vi "rx_trig_capt.vi"(7 "number of samples":i64=-1, 8 "error in (no error)":errorcluster, 9 "reference\nposition":dbl format="%0.2f", 10 "trigger level":dbl format="%0.2f", 11 "session handle":refnum<k15>) -> (0 "error out":errorcluster, 1 "packet found":bool, 2 "IQ Waveform":cluster{"t0":dbl, "dt":dbl, "Y":cdb[]}, 3 "session handle out":refnum<k15>)   [LabVIEW 2012, in "gds_hw_config.lvlib"]
uses:
  <instrlib>/niUSRP/niUSRP Fetch Rx Data (CDB Cluster).vi
  gds_hw_config.lvlib
  <vilib>/Analysis/NI_AALPro.lvlib
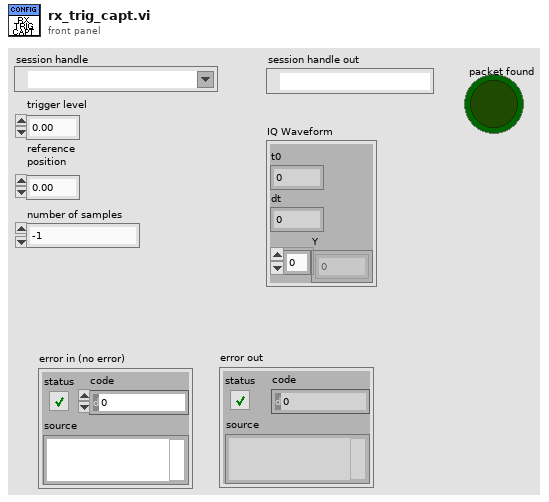
[diagram p1: front panel]
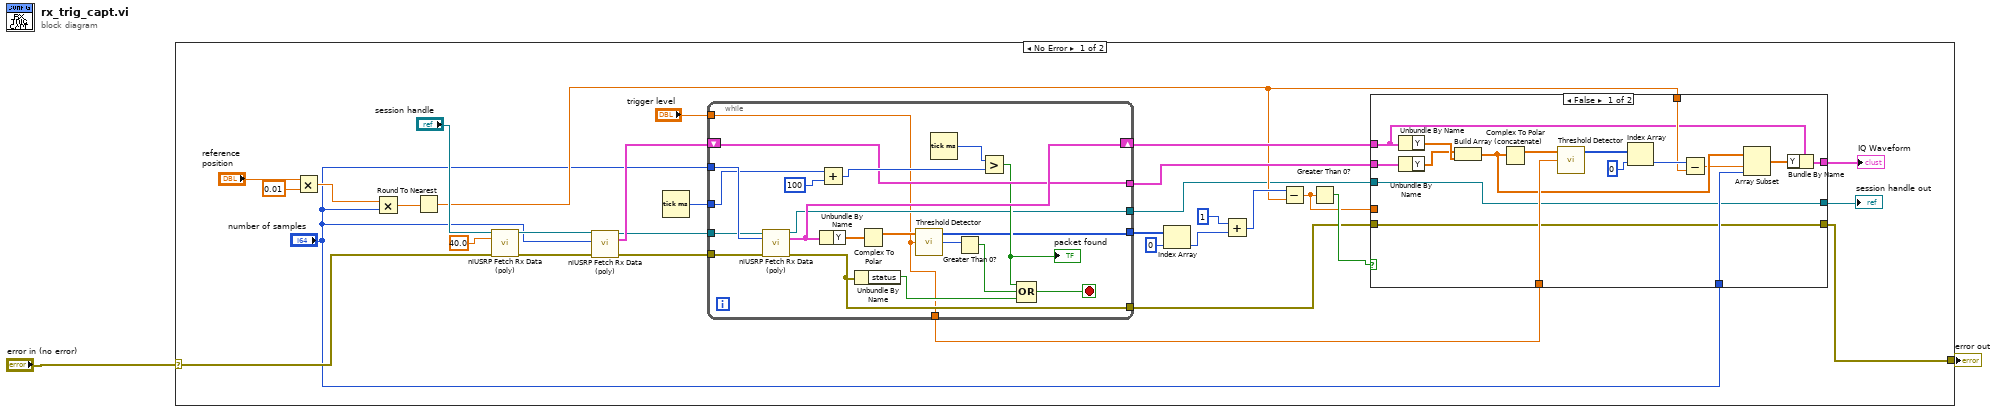
[diagram p0: block diagram]
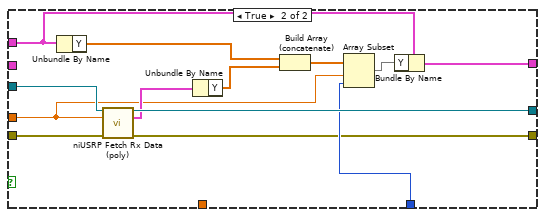
[diagram p2: hidden frame]
diagram:
  n1 = case shown="No Error" "error in (no error)" {
    selector: "error in (no error)" -> [w28 w84]
    tunnel: [w4 w84] -> w1
    frame No Error {
      n2 = Multiply(x="reference\nposition", y=0.01) -> (x*y=w31:dbl)
      n3 = Multiply(x=w31, y="number of samples") -> (x*y=w30:dbl)
      n4 = Round To Nearest(number=w30) -> (nearest integer value=w10:dbl)
      n5 = call-poly <instrlib>:"niUSRP Fetch Rx Data (poly).vi"("session handle"="session handle", "number of samples"=40.0 ("timeout"), "error in (no error)"=w28) -> ("session handle out"=w26:refnum<k15>, "error out"=w25:errorcluster)  [unwired: 9 in, 2 out]
      n6 = call-poly <instrlib>:"niUSRP Fetch Rx Data (poly).vi"("session handle"=w26, "number of samples"="number of samples", "error in (no error)"=w25) -> ("session handle out"=w22:refnum<k15>, "data"=w24:cluster{"t0":dbl, "dt":dbl, "Y":cdb[]}, "error out"=w23:errorcluster)  [unwired: 9 in, 1 out]
      n7 = Tick Count (ms)() -> (millisecond timer value=w21:u32)
      n8 = while {
        shift-right: [w76] -> w13
        shift-left: w24 -> [w72]
        tunnel: w23 -> [w83]
        tunnel: "number of samples" -> [w82]
        tunnel: w22 -> [w81]
        tunnel: w21 -> [w80]
        tunnel: "trigger level" -> [w64]
        tunnel: [w72] -> w12
        tunnel: [w67] -> w19
        tunnel: [w66] -> w7
        tunnel: [w65] -> w5
        tunnel: [w64] -> w11
        stop <- w69 stop-if-true
        n9 = call-poly <instrlib>:"niUSRP Fetch Rx Data (poly).vi"("session handle"=w81, "number of samples"=w82, "error in (no error)"=w83) -> ("session handle out"=w66:refnum<k15>, "data"=w76:cluster{"t0":dbl, "dt":dbl, "Y":cdb[]}, "error out"=w65:errorcluster)  [unwired: 9 in, 1 out]
        n10 = Add(x=w80, y=u32 100) -> (x+y=w74:u32)
        n11 = Unbundle By Name(w76) -> ("Y"=w78:cdb[])
        n12 = Unbundle By Name(w65) -> ("status"=w70:bool)
        n13 = Complex To Polar(r * e^(i*theta)=w78) -> (r=w77:dbl[])  [unwired: 1 out]
        n14 = call <vilib>:"Threshold Detector.vi"("threshold"=w64, "X"=w77) -> ("count"=w75:i32, "Indices"=w67:i32[])  [unwired: 1 in, 1 out]
        n15 = Tick Count (ms)() -> (millisecond timer value=w73:u32)
        n16 = Greater Than 0?(x=w75) -> (x > 0?=w71:bool)
        n17 = Greater?(x=w73, y=w74) -> (0:w68:bool)
        "packet found" <- w68
        n18 = Compound Arithmetic op=OR(w68, w71, w70) -> (w69:bool)
      }
      n19 = Index Array(array=w19, index=0) -> (element=w17:i32)
      n20 = Add(x=1, y=w17) -> (x+y=w15:i32)
      n21 = Subtract(x=w15, y=w10) -> (x-y=w3:dbl)
      n22 = Greater Than 0?(x=w3) -> (x > 0?=w14:bool)
      n23 = case shown="False" w14 {
        tunnel: w13 -> [w37 w53]
        tunnel: w12 -> [w50 _]
        tunnel: w11 -> [w46 _]
        tunnel: w10 -> [w42 _]
        tunnel: "number of samples" -> [w39 w56]
        tunnel: [w36 w52] -> w8
        tunnel: w7 -> [w35 w62]
        tunnel: [w35 w61] -> w6
        tunnel: w5 -> [w34 w63]
        tunnel: [w34 w51] -> w4
        tunnel: w3 -> [_ w55]
        frame False {
          n24 = Unbundle By Name(w37) -> ("Y"=w49:cdb[])
          n25 = Unbundle By Name(w50) -> ("Y"=w48:cdb[])
          n26 = Build Array (concatenate)(w48, w49) -> (w41:cdb[])
          n27 = Complex To Polar(r * e^(i*theta)=w41) -> (r=w47:dbl[])  [unwired: 1 out]
          n28 = call <vilib>:"Threshold Detector.vi"("threshold"=w46, "X"=w47) -> ("Indices"=w44:i32[])  [unwired: 1 in, 2 out]
          n29 = Index Array(array=w44, index=0) -> (element=w43:i32)
          n30 = Subtract(x=w43, y=w42) -> (x-y=w40:dbl)
          n31 = Array Subset(array=w41, index=w40, length=w39) -> (w38:cdb[])
          n32 = Bundle By Name(cluster=w37, "Y"=w38) -> (w36:cluster{"t0":dbl, "dt":dbl, "Y":cdb[]})
        }
        frame True {
          n33 = Unbundle By Name(w53) -> ("Y"=w58:cdb[])
          n34 = call-poly <instrlib>:"niUSRP Fetch Rx Data (poly).vi"("session handle"=w62, "number of samples"=w55, "error in (no error)"=w63) -> ("session handle out"=w61:refnum<k15>, "data"=w60:cluster{"t0":dbl, "dt":dbl, "Y":cdb[]}, "error out"=w51:errorcluster)  [unwired: 9 in, 1 out]
          n35 = Unbundle By Name(w60) -> ("Y"=w59:cdb[])
          n36 = Build Array (concatenate)(w58, w59) -> (w57:cdb[])
          n37 = Array Subset(array=w57, index=w55, length=w56) -> (w54:cdb[])
          n38 = Bundle By Name(cluster=w53, "Y"=w54) -> (w52:cluster{"t0":dbl, "dt":dbl, "Y":cdb[]})
        }
      }
      "IQ Waveform" <- w8
      "session handle out" <- w6
    }
    frame Error {
    }
  }
  "error out" <- w1
